vi "write_timing_array.vi"(4 "error in":errorcluster, 5 "delay array":dbl[](array[numeric]), 7 "VISA resource in":refnum<visa-resource-name>) -> (0 "error out 2":errorcluster, 3 "VISA resource out":refnum<visa-resource-name>)   [LabVIEW 2011]
doc: "Reads all delay values stored in the DG645 and returns them in an array, from t0 to H.\nSee DG645 documentation for mor info."
panel:
  out "Array":string[](array[string])
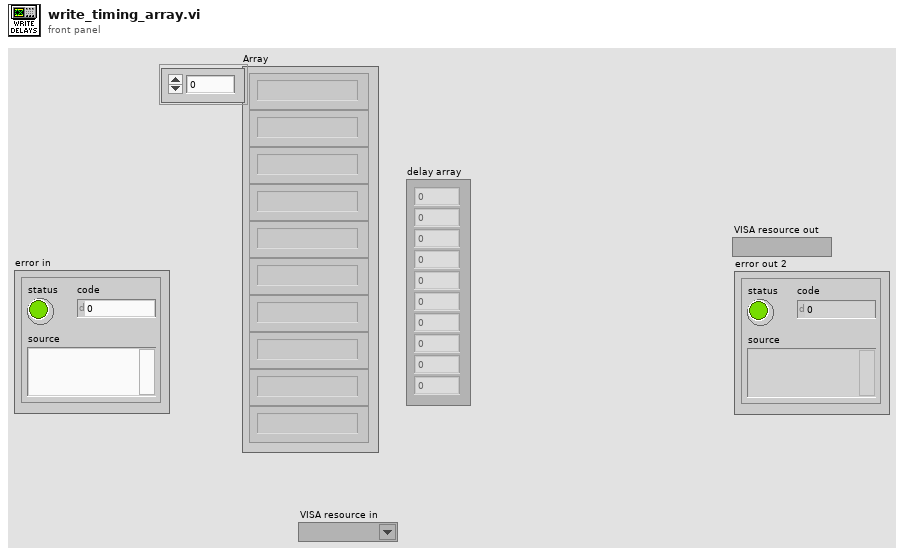
[diagram p1: front panel]
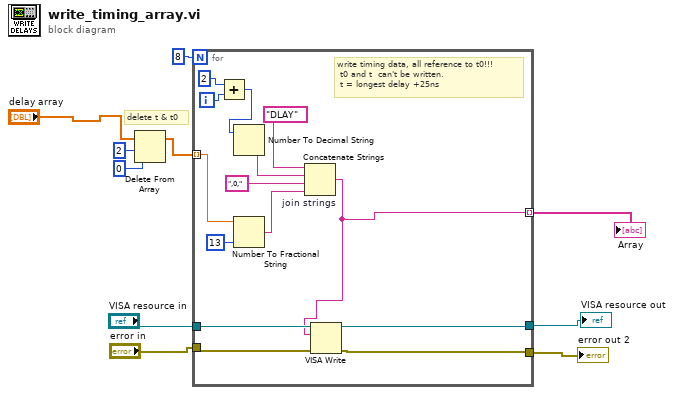
[diagram p0: block diagram]
diagram:
  # "delete t & t0"
  n1 = Delete From Array(array="delay array", length=2, index=0) -> (array with subset deleted=w2:dbl[])  [unwired: 1 out]
  n2 = for {
    N: 8 -> [_]
    tunnel: "error in" -> [w22]
    tunnel: [w23] -> w6
    tunnel: "VISA resource in" -> [w19]
    tunnel: [w24] -> w7
    tunnel: [w15] -> w5 mode=indexing
    tunnel: w2 -> [w14] mode=indexing
    i -> [w17]
    # "write timing data, all reference to t0!!!\n t0 and t  can't be written.\n t = longest delay +25ns"
    n3 = Add(x=2, y=w17) -> (x+y=w12:i32)
    n4 = Number To Decimal String(number=w12) -> (decimal integer string=w20:string)  [unwired: 1 in]
    n5 = Number To Fractional String(number=w14, precision (6)=i16 13) -> (F-format string=w16:string)  [unwired: 2 in]
    n6 = Concatenate Strings "join strings"("DLAY" ("string"), w20, ",0," ("string"), w16) -> (w15:string)
    n7 = VISA Write(VISA resource name=w19, write buffer=w15, error in (no error)=w22) -> (VISA resource name out=w24:refnum<visa-resource-name>, error out=w23:errorcluster)  [unwired: 1 out]
  }
  "VISA resource out" <- w7
  "error out 2" <- w6
  "Array" <- w5
